vi "start.vi"(8 "error in (no error)":errorcluster, 11 "Counter in":refnum<class "Counter.lvclass">) -> (0 "error out":errorcluster, 3 "Counter out":refnum<class "Counter.lvclass">)   [LabVIEW 2014, in "Counter.lvclass"]
uses:
  Counter.lvclass
  Counter.lvclass/Counter.ctl
  Globals.vi
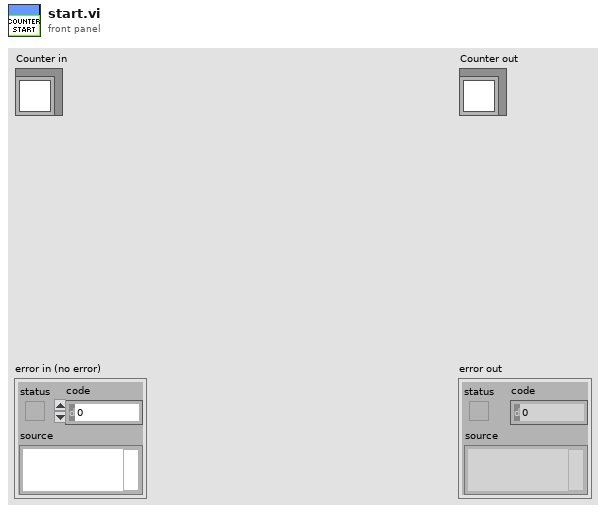
[diagram p1: front panel]
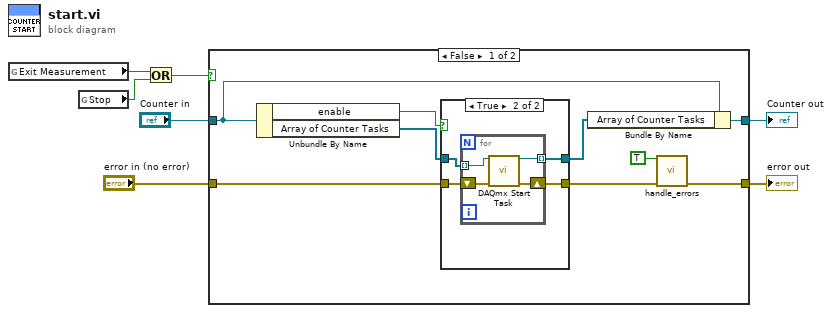
[diagram p0: block diagram]
diagram:
  n1 = global read "Globals.vi" "Exit Measurement"() -> (w3:bool)
  n2 = global read "Globals.vi" "Stop"() -> (w4:bool)
  n3 = Or(x=w3, y=w4) -> (x .or. y?=w2:bool)
  n4 = case shown="False" w2 {
    tunnel: [w9 w27] -> w5
    tunnel: [w13 w28] -> w6
    tunnel: "Counter in" -> [w14 w28]
    tunnel: "error in (no error)" -> [w8 w27]
    frame False {
      n5 = Unbundle By Name(w14) -> ("enable"=w16:bool, "Array of Counter Tasks"=w15:refnum<k21>[])
      n6 = case shown="True" w16 {
        tunnel: w15 -> [w18 w22]
        tunnel: [w17 w21] -> w11
        tunnel: [w18 w20] -> w12
        tunnel: w8 -> [w17 w19]
        frame False {
        }
        frame True {
          n7 = for {
            tunnel: w22 -> [w26] mode=indexing
            shift-right: [w24] -> w21
            shift-left: w19 -> [w25]
            tunnel: [w23] -> w20 mode=indexing
            n8 = call <vilib>:"DAQmx Start Task.vi"("task/channels in"=w26, "error in"=w25) -> ("task out"=w23:refnum<k21>, "error out"=w24:errorcluster)  [unwired: 12 in]
          }
        }
      }
      n9 = Bundle By Name(cluster=w14, "Array of Counter Tasks"=w12) -> (w13:refnum<class "Counter.lvclass">)
      n10 = call "handle_errors.vi"("Exit Operation"=TRUE ("Exit Measurement"), "error in (no error)"=w11) -> ("error out"=w9:errorcluster)  [unwired: 13 in]
    }
    frame True {
    }
  }
  "error out" <- w5
  "Counter out" <- w6
